vi "svfa_Average Array (real).vi"(6 "averages completed in":dbl, 7 "processing control":T1(ring), 8 "number of averages":u32, 9 "weighting mode":enum16{"Linear", "Exponential"}(ring), 10 "previous average array":dbl[](array[numeric]) format="%.2p", 11 "array":dbl[](array[numeric]) format="%.2p") -> (1 "averaging done":bool, 2 "averages completed out":dbl, 3 "average array":dbl[](array[numeric]) format="%.2p")   [LabVIEW 2017]
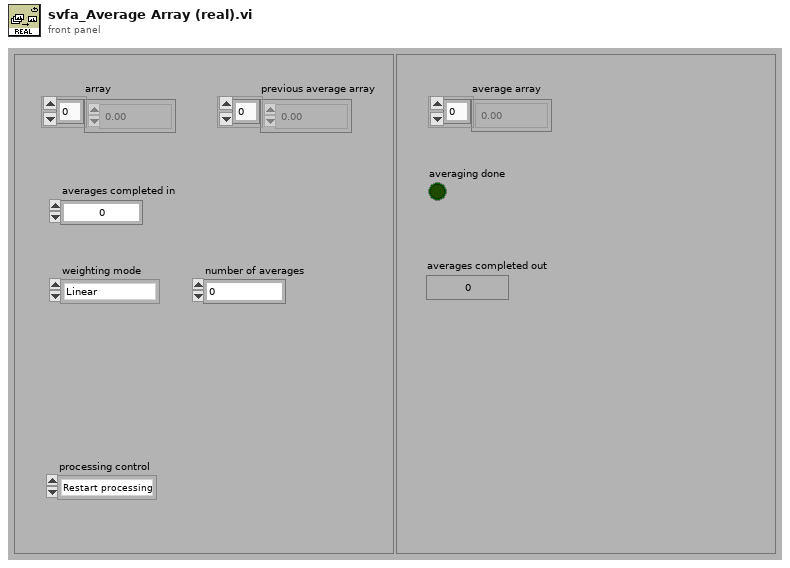
[diagram p1: front panel]
types:
  T1 = enum16{"Restart processing", "Continue processing", "Skip processing"}
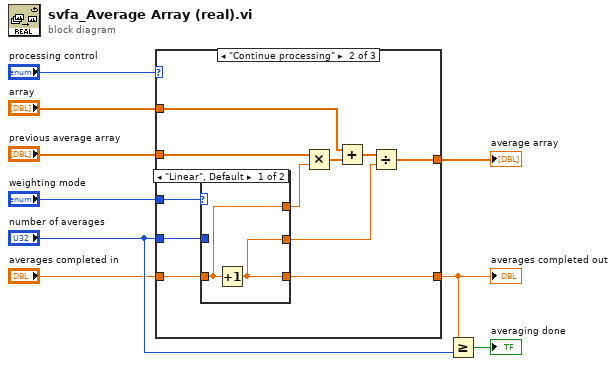
[diagram p0: block diagram]
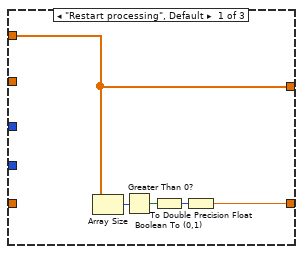
[diagram p2: hidden frame]
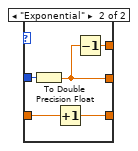
[diagram p3: hidden frame]
diagram:
  n1 = case shown="\"Continue processing\"" "processing control" {
    tunnel: [w10 w23 w34] -> w5
    tunnel: "number of averages" -> [_ w20 _]
    tunnel: "weighting mode" -> [_ w19 _]
    tunnel: "averages completed in" -> [_ w18 w34]
    tunnel: "previous average array" -> [_ w17 w33]
    tunnel: "array" -> [w14 w16 _]
    tunnel: [w14 w15 w33] -> w3
    frame "Restart processing", Default {
      n2 = Array Size(array=w14) -> (size(s)=w13:i32)
      n3 = Greater Than 0?(x=w13) -> (x > 0?=w12:bool)
      n4 = Boolean To (0,1)(Boolean=w12) -> (0, 1=w11:i16)
      n5 = To Double Precision Float(number=w11) -> (double precision float=w10:dbl)
    }
    frame "Continue processing" {
      n6 = case shown="\"Linear\", Default" w19 {
        tunnel: w18 -> [w27 w31]
        tunnel: [w26 w32] -> w23
        tunnel: [w27 w28] -> w24
        tunnel: [w26 w29] -> w22
        tunnel: w20 -> [_ w30]
        frame "Linear", Default {
          n7 = Increment(x=w27) -> (x+1=w26:dbl)
        }
        frame "Exponential" {
          n8 = To Double Precision Float(number=w30) -> (double precision float=w29:dbl)
          n9 = Increment(x=w31) -> (x+1=w32:dbl)
          n10 = Decrement(x=w29) -> (x-1=w28:dbl)
        }
      }
      n11 = Multiply(x=w17, y=w24) -> (x*y=w21:dbl[])
      n12 = Add(x=w16, y=w21) -> (x+y=w25:dbl[])
      n13 = Divide(x=w25, y=w22) -> (x/y=w15:dbl[])
    }
    frame "Skip processing" {
    }
  }
  "averages completed out" <- w5
  "average array" <- w3
  n14 = Greater Or Equal?(x=w5, y="number of averages") -> (x >= y?=→"averaging done":bool)
